vi "Subvi Setup Lamp And Exposure.vi"(0 "PassImageType":u8) -> ()   [LabVIEW 2012]
uses:
  ProSCI Global.vi
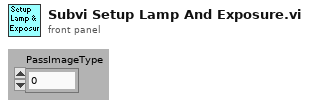
[diagram p1: front panel]
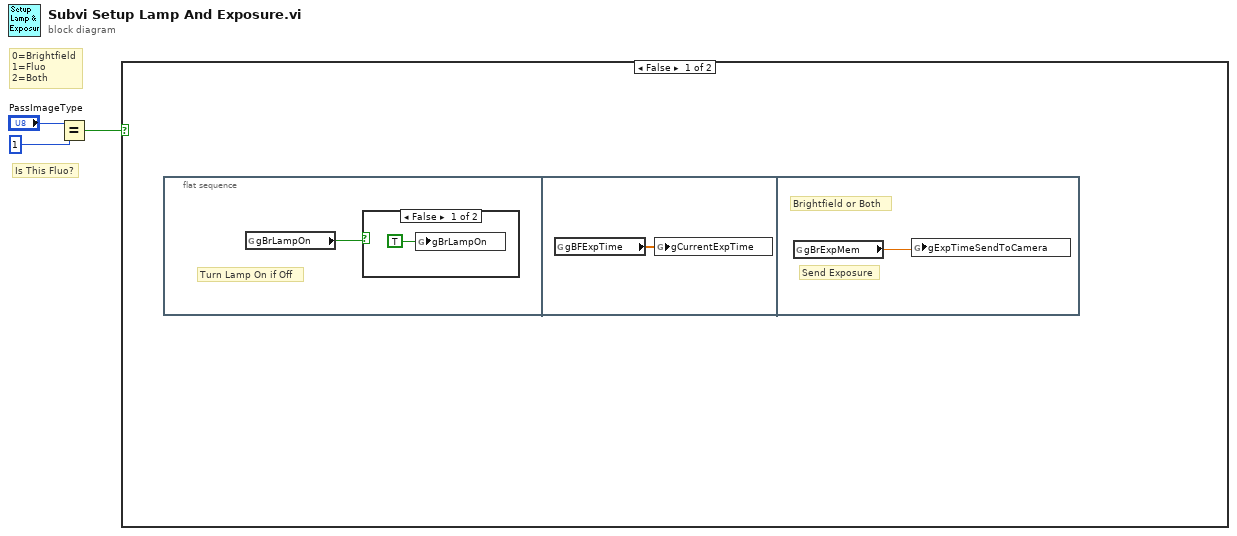
[diagram p0: block diagram]
diagram:
  # "Is This Fluo?"
  # "0=Brightfield\n1=Fluo\n2=Both"
  n1 = Equal?(x="PassImageType", y=u8 1) -> (x = y?=w1:bool)
  n2 = case shown="False" w1 {
    frame False {
      n3 = flat-sequence {
        frame #0 {
          # "Turn Lamp On if Off"
          n4 = global read "ProSCI Global.vi" "gBrLampOn"() -> (w4:bool)
          n5 = case shown="False" w4 {
            frame False {
              n6 = global write "ProSCI Global.vi" "gBrLampOn"(TRUE ("gBrLampOn")) -> ()
            }
            frame True {
            }
          }
        }
        frame #1 {
          n7 = global read "ProSCI Global.vi" "gBFExpTime"() -> (w6:dbl[])
          n8 = global write "ProSCI Global.vi" "gCurrentExpTime"(w6) -> ()
        }
        frame #2 {
          # "Send Exposure"
          # "Brightfield or Both"
          n9 = global read "ProSCI Global.vi" "gBrExpMem"() -> (w7:dbl)
          n10 = global write "ProSCI Global.vi" "gExpTimeSendToCamera"(w7) -> ()
        }
      }
    }
    frame True {
      # "Move to Imaging subvi!!!"
    }
  }
